vi "fileReader.vi"(8 "error in":errorcluster, 11 "filepath":path) -> (0 "error out":errorcluster, 3 "dataout":u32[](array[numeric]) format="%x")   [LabVIEW 2014]
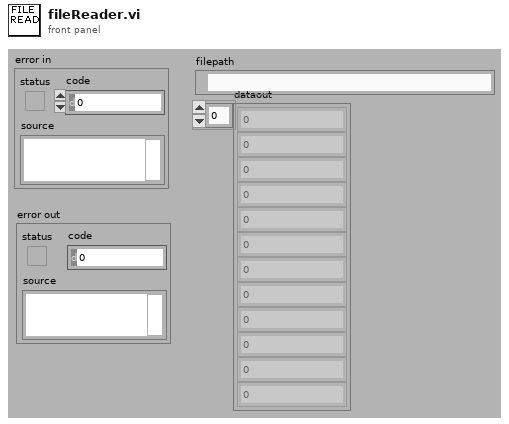
[diagram p1: front panel]
types:
  T1 = enum16{"big-endian, network order", "native, host order", "little-endian"}
  T2 = enum16{"open", "replace", "create", "open or create", "replace or create", "replace or create with confirmation"}
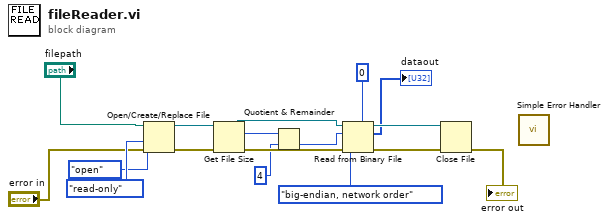
[diagram p0: block diagram]
diagram:
  n1 = Open/Create/Replace File(file path (use dialog)="filepath", error in="error in", operation (0:open)=T2."open", access (0:read/write)=enum16{"read/write", "read-only", "write-only"}."read-only") -> (refnum out=w6:refnum<file>, error out=w8:errorcluster)  [unwired: 3 out]
  n2 = Get File Size(file=w6, error in=w8) -> (refnum out=w5:refnum<file>, size (in bytes)=w4:i64, 0:w7:errorcluster)
  n3 = Quotient & Remainder(x=w4, y=i64 4) -> (floor(x/y)=w3:i64)  [unwired: 1 out]
  n4 = Read from Binary File(5:u32 0 ("data type"), 8:w7, 9:T1."big-endian, network order" ("byte order (0:big-endian, network order)"), 10:w3, 11:w5) -> (0:w12:errorcluster, 2:→"dataout":u32[], 3:w13:refnum<file>)  [unwired: 2 out]
  n5 = Close File(refnum=w13, error in=w12) -> (error out=→"error out":errorcluster)  [unwired: 1 out]
  n6 = call <vilib>:"Simple Error Handler.vi"() -> ()  [unwired: 2 in, 8 out]
